vi "getRegisters.vi"(0 "AddressSpace in":refnum<class "AddressSpace.lvclass">) -> (4 "AddressSpace out":refnum<class "AddressSpace.lvclass">, 6 "settingsReg":T2={"numberOfInterleaves"="", "rampRate"="", "manualInput"="", "perturbAmp"="", "perturbAngleInc"="", "reset"="", "state"="", "gains"="", "Currents"="Currents"}, 8 "modRegisters":T1={"numberOfInterleaves"="Register", "Enable"="Register", "triangleInc"="Register", "Deadband"="Register", "Enabled"="Register"})   [LabVIEW 2017, in "BuckBoost.lvlib" / "AddressSpace.lvclass"]
uses:
  AddressSpace.lvclass
  contSettings.ctl
  modRegisters.ctl
  AddressSpace.lvclass/AddressSpace.ctl
  BuckBoost.lvlib
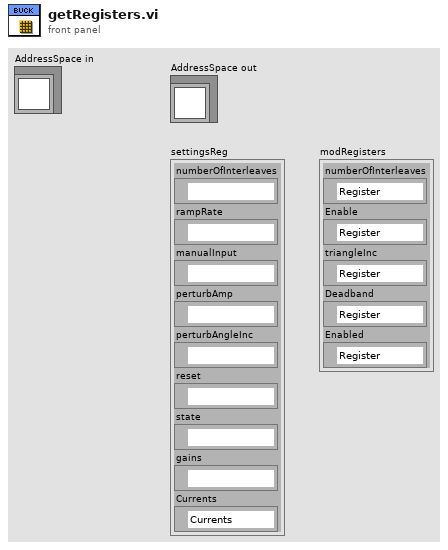
[diagram p1: front panel]
types:
  T1 = typedef "BuckBoost.lvlib/modRegisters.ctl" = cluster{"numberOfInterleaves":refnum<k21>, "Enable":refnum<k21>, "triangleInc":refnum<k21>, "Deadband":refnum<k21>, "Enabled":refnum<k21>}
  T2 = typedef "BuckBoost.lvlib/contSettings.ctl" = cluster{"numberOfInterleaves":refnum<k21>, "rampRate":refnum<k21>, "manualInput":refnum<k21>, "perturbAmp":refnum<k21>, "perturbAngleInc":refnum<k21>, "reset":refnum<k21>, "state":refnum<k21>, "gains":refnum<k21>, "Currents":refnum<k21>}
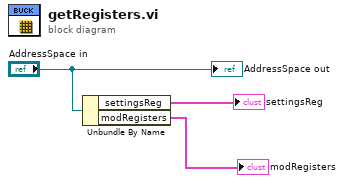
[diagram p0: block diagram]
diagram:
  n1 = Unbundle By Name("AddressSpace in") -> ("settingsReg"=→"settingsReg":T2, "modRegisters"=→"modRegisters":T1)
  "AddressSpace out" <- "AddressSpace in"
